vi "Send Message.vi"(8 "error in (no error)":errorcluster, 10 "Message":string, 11 "Channel GUI in":refnum<class "Channel GEI.lvclass">) -> (0 "error out":errorcluster, 3 "Channel GUI out":refnum<class "Channel GEI.lvclass">)   [LabVIEW 2018, in "Channel GEI.lvclass"]
uses:
  Channel GEI.lvclass
  Channel GEI.lvclass/Channel GEI.ctl
  RxTx/RxTx.lvclass
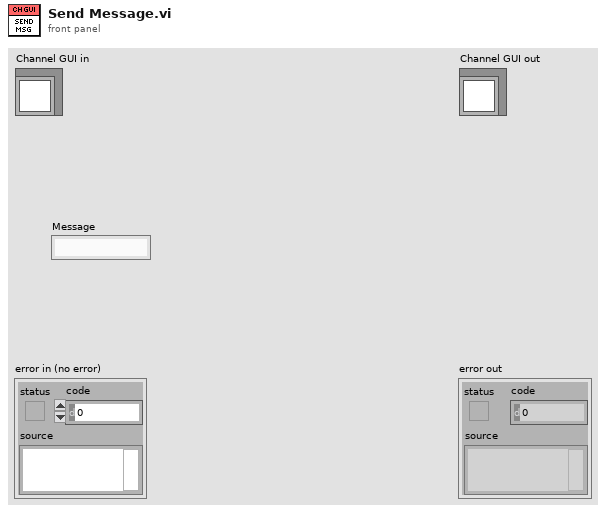
[diagram p1: front panel]
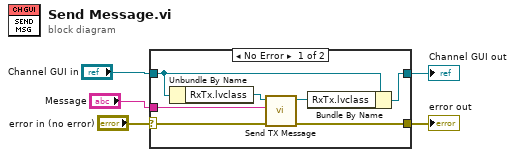
[diagram p0: block diagram]
diagram:
  n1 = case shown="No Error" "error in (no error)" {
    selector: "error in (no error)" -> [w11 w14]
    tunnel: [w12 w14] -> w4
    tunnel: [w8 w13] -> w2
    tunnel: "Channel GUI in" -> [w9 w13]
    tunnel: "Message" -> [w6 _]
    frame No Error {
      n2 = Unbundle By Name(w9) -> ("RxTx.lvclass"=w10:refnum<class "RxTx.lvclass">)
      n3 = call "Send TX Message.vi"("error in (no error)"=w11, "element"=w6, "RxTx in"=w10) -> ("error out"=w12:errorcluster, "RxTx out"=w7:refnum<class "RxTx.lvclass">)  [unwired: 7 in]
      n4 = Bundle By Name(cluster=w9, "RxTx.lvclass"=w7) -> (w8:refnum<class "Channel GEI.lvclass">)
    }
    frame Error {
    }
  }
  "error out" <- w4
  "Channel GUI out" <- w2
